vi "Fpga-Top-Level.vi"() -> ()   [LabVIEW 2015]
uses:
  SETI_LV_FPGA/SETI_LV_FPGA.lvclass
  SETI_LV/SETI_LV.lvlib
panel:
  out "error out":errorcluster
  out "Errors":cluster{"lower limit":sgl, "Index":i32}[](array[cluster])
  out "Results\nMatch?":bool
  in  "Max Error":sgl=0.0001
  out "Expected\nPower Spectrum":sgl[](array[numeric])
  in  "error in":errorcluster
  in  "Run #\nto Load":i32=1
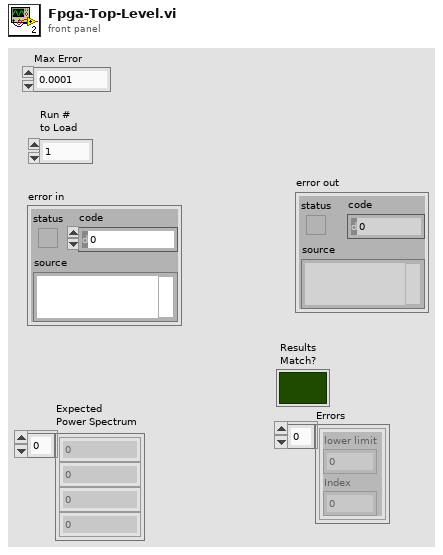
[diagram p1: front panel]
types:
  T1 = typedef "SETI_LV.lvlib/ChirpFFT Pairs.ctl" = cluster{"Chirp/Fft Pair 1 - Chirp Rate":dbl, "Chirp/Fft Pair 1 - Chirp Rate Ind":i32, "Chirp/Fft Pair 1 - Fft Length":i32, "Chirp/Fft Pair 1 - Pulse Find":i32, "Chirp/Fft Pair 1 - Gauss Fit":i32}
  T2 = typedef "SETI_LV.lvlib/Power Spectrum Data.ctl" = cluster{"icfft":i32, "NumDataPoints":i32, "Power Spectrum":sgl[]}
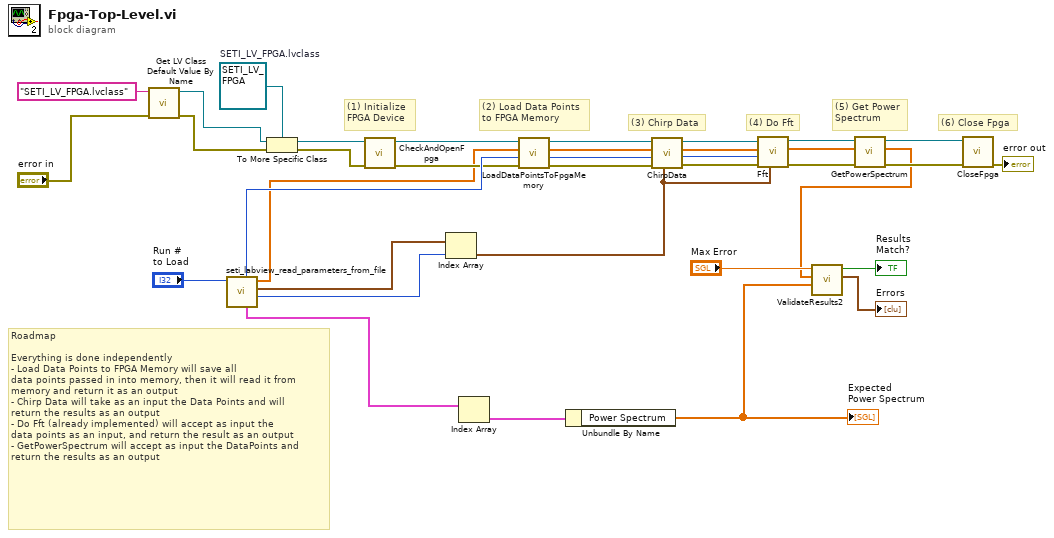
[diagram p0: block diagram]
diagram:
  w36 = refnum<class "SETI_LV_FPGA.lvclass"> refnum  # SETI_LV_FPGA.lvclass
  # "(6) Close Fpga"
  # "(5) Get Power\nSpectrum"
  # "Roadmap\n\nEverything is done independently\n- Load Data Points to FPGA Memory will save all\ndata points passed in into memory, then it will read it from\nmemory and return it as an output\n- Chirp Data will take as an input the Data Points and will\nreturn the results as an output\n- Do Fft (already implemented) will accept as input the\ndata points as an input, and return the result as an output\n- GetPowerSpectrum will accept as input the DataPoints and\nreturn the results as an output"
  # "(4) Do Fft"
  # "(3) Chirp Data"
  # "(1) Initialize\nFPGA Device"
  # "(2) Load Data Points\nto FPGA Memory"
  n1 = call <vilib>:"Get LV Class Default Value By Name.vi"("error in (no error)"="error in", "class name"="SETI_LV_FPGA.lvclass") -> ("error out"=w10:errorcluster, "object"=w12:refnum<class>)  [unwired: 8 in]
  n2 = call "seti_labview_read_parameters_from_file.vi"("Run Number\nto Load"="Run #\nto Load") -> ("start_icfft"=w9:i32, "Chirp FFT Pairs"=w14:T1[], "Data Points (Source)"=w25:csg[], "Array of Power Spectrum Data\n(Expected Results)"=w7:T2[], "NumDataPoints"=w34:u32)  [unwired: 4 in, 2 out]
  n3 = To More Specific Class(target class=w36, reference=w12, error in=w10) -> (specific class reference=w33:refnum<class "SETI_LV_FPGA.lvclass">, error out=w30:errorcluster)
  n4 = call-dynamic "CheckAndOpenFpga.vi"("error in (no error)"=w30, "SETI_LV_FPGA in"=w33) -> ("error out"=w31:errorcluster, "SETI_LV_FPGA out"=w32:refnum<class "SETI_LV_FPGA.lvclass">)  [unwired: 8 in]
  n5 = Index Array(array=w14, index=w9) -> (element=w13:T1)
  n6 = Index Array(array=w7) -> (element=w8:T2)  [unwired: 1 in]
  n7 = call-dynamic "LoadDataPointsToFpgaMemory.vi"("error in (no error)"=w31, "NumDataPoints"=w34, "Work Unit Data Points"=w25, "SETI_LV_FPGA in"=w32) -> ("error out"=w29:errorcluster, "NumDataPoints"=w23:u32, "Work Unit Data Points"=w24:csg[], "SETI_LV_FPGA out"=w28:refnum<class "SETI_LV_FPGA.lvclass">)  [unwired: 4 in]
  n8 = Unbundle By Name(w8) -> ("Power Spectrum"=w3:sgl[])
  "Expected\nPower Spectrum" <- w3
  n9 = call-dynamic "ChirpData.vi"("element"=w13, "error in (no error)"=w29, "NumDataPoints"=w23, "Work Unit Data Points"=w24, "SETI_LV_FPGA in"=w28) -> ("error out"=w26:errorcluster, "NumDataPoints"=w21:u32, "ChirpedData out"=w22:csg[], "SETI_LV_FPGA out"=w27:refnum<class "SETI_LV_FPGA.lvclass">)  [unwired: 3 in]
  n10 = call-dynamic "Fft.vi"("Chirp Parameters (in)"=w13, "error in (no error)"=w26, "NumDataPoints"=w21, "ChirpedData in"=w22, "SETI_LV_FPGA in"=w27) -> ("error out"=w18:errorcluster, "FftData out"=w19:csg[], "SETI_LV_FPGA out"=w20:refnum<class "SETI_LV_FPGA.lvclass">)  [unwired: 3 in, 1 out]
  n11 = call-dynamic "GetPowerSpectrum.vi"("error in (no error)"=w18, "FftData in"=w19, "SETI_LV_FPGA in"=w20) -> ("error out"=w16:errorcluster, "PowerSpectrum out"=w2:sgl[], "SETI_LV_FPGA out"=w17:refnum<class "SETI_LV_FPGA.lvclass">)  [unwired: 6 in]
  n12 = call "ValidateResults2.vi"("PowerSpectrum2 (in)"=w3, "PowerSpectrum1 (in)"=w2, "Max Error"="Max Error") -> ("Errors"=→"Errors":cluster{"lower limit":sgl, "Index":i32}[], "Results Match?"=→"Results\nMatch?":bool)  [unwired: 7 in]
  n13 = call-dynamic "CloseFpga.vi"("error in (no error)"=w16, "SETI_LV_FPGA in"=w17) -> ("error out"=→"error out":errorcluster)  [unwired: 8 in, 1 out]
